vi "How Many Steps.vi"(4 "Step":dbl, 6 "Add step back":bool, 7 "Increment mode":T1, 9 "Number of steps":i32, 10 "End":dbl, 11 "Start":dbl) -> (1 "Step out":dbl, 2 "Number of steps out":i32, 3 "Start out":dbl)   [LabVIEW 2021]
uses:
  Increment mode.ctl
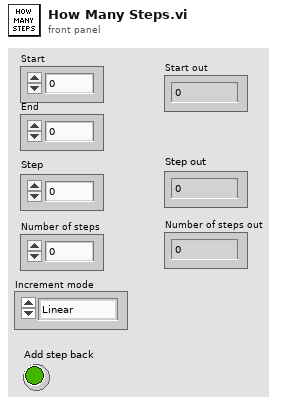
[diagram p1: front panel]
types:
  T1 = typedef "Increment mode.ctl" = enum16{"Linear", "Square root", "Square", "Log", "Exponent"}
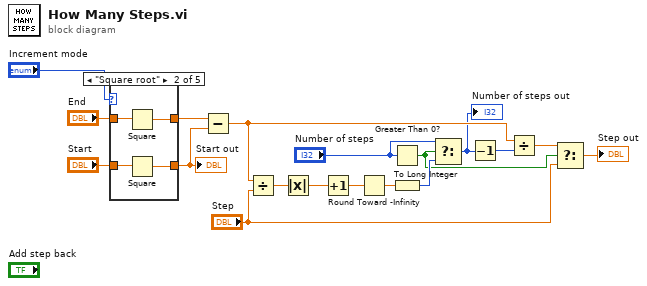
[diagram p0: block diagram]
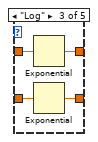
[diagram p3: hidden frame]
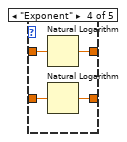
[diagram p4: hidden frame]
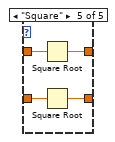
[diagram p5: hidden frame]
diagram:
  n1 = case shown="\"Square root\"" "Increment mode" {
    tunnel: [w20 w24 w28 w32 w36] -> w18
    tunnel: "End" -> [w20 w23 w27 w31 w35]
    tunnel: "Start" -> [w19 w22 w26 w30 w34]
    tunnel: [w19 w21 w25 w29 w33] -> w1
    frame "Linear", Default {
    }
    frame "Square root" {
      n2 = Square(x=w23) -> (x^2=w24:dbl)
      n3 = Square(x=w22) -> (x^2=w21:dbl)
    }
    frame "Log" {
      n4 = Exponential(1:w27) -> (0:w28:dbl)
      n5 = Exponential(1:w26) -> (0:w25:dbl)
    }
    frame "Exponent" {
      n6 = Natural Logarithm(1:w31) -> (0:w32:dbl)
      n7 = Natural Logarithm(1:w30) -> (0:w29:dbl)
    }
    frame "Square" {
      n8 = Square Root(x=w35) -> (sqrt(x)=w36:dbl)
      n9 = Square Root(x=w34) -> (sqrt(x)=w33:dbl)
    }
  }
  "Start out" <- w1
  n10 = Subtract(x=w18, y=w1) -> (x-y=w12:dbl)
  n11 = Divide(x=w12, y="Step") -> (x/y=w13:dbl)
  n12 = Absolute Value(x=w13) -> (abs(x)=w16:dbl)
  n13 = Increment(x=w16) -> (x+1=w14:dbl)
  n14 = Round Toward -Infinity(1:w14) -> (0:w15:dbl)
  n15 = Greater Than 0?(x="Number of steps") -> (x > 0?=w10:bool)
  n16 = To Long Integer(number=w15) -> (32bit integer=w11:i32)
  n17 = Select(t="Number of steps", s=w10, f=w11) -> (s? t:f=w2:i32)
  "Number of steps out" <- w2
  n18 = Decrement(x=w2) -> (x-1=w17:i32)
  n19 = Divide(x=w12, y=w17) -> (x/y=w9:dbl)
  n20 = Select(t=w9, s=w10, f="Step") -> (s? t:f=→"Step out":dbl)
